vi "UniqueID2StatID.vi"(11 "UniqueID":string) -> (3 "StatID":string)   [LabVIEW 2013]
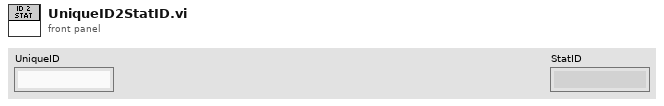
[diagram p1: front panel]
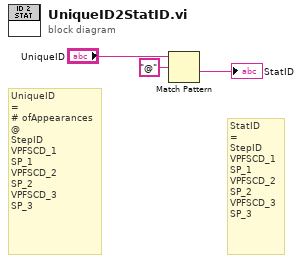
[diagram p0: block diagram]
diagram:
  # "StatID\n=\nStepID\nVPFSCD_1\nSP_1\nVPFSCD_2\nSP_2\nVPFSCD_3\nSP_3"
  # "UniqueID\n=\n# ofAppearances\n@\nStepID\nVPFSCD_1\nSP_1\nVPFSCD_2\nSP_2\nVPFSCD_3\nSP_3"
  n1 = Match Pattern(string="UniqueID", regular expression="@") -> (after substring=→"StatID":string)  [unwired: 1 in, 3 out]
